vi "Flatten Multi D Arrays.vi"() -> ()   [LabVIEW 2011]
uses:
  JSON Scalar/variants/Variant Data Typdef.ctl
  <vilib>/Utility/VariantDataType/Type.ctl
  JSON Scalar/JSON Scalar.lvclass
  <vilib>/Utility/VariantDataType/VariantType.lvlib
panel:
  out "dimensions?":bool
  out "# 3D Array Dimensions":i32[](array[numeric])=[4, 3, 3]
  out "3D Variant Data":T1[](array[typedef])=[{"Type Enum"=enum."Double Float", "Name"="", "Variant"=variant(dbl 1.0)}, {"Type Enum"=enum."Double Float", "Name"="", "Variant"=variant(dbl 2.0)}, {"Type Enum"=enum."Double Float", "Name"="", "Variant"=variant(dbl 3.0)}, {"Type Enum"=enum."Double Float", "Name"="", "Variant"=variant(dbl 4.0)}, {"Type Enum"=enum."Double Float", "Name"="", "Variant"=variant(dbl 5.0)}, {"Type Enum"=enum."Double Float", "Name"="", "Variant"=variant(dbl 6.0)}, {"Type Enum"=enum."Double Float", "Name"="", "Variant"=variant(dbl 7.0)}, {"Type Enum"=enum."Double Float", "Name"="", "Variant"=variant(dbl 8.0)}, {"Type Enum"=enum."Double Float", "Name"="", "Variant"=variant(dbl 9.0)}, {"Type Enum"=enum."Double Float", "Name"="", "Variant"=variant(dbl 10.0)}, {"Type Enum"=enum."Double Float", "Name"="", "Variant"=variant(dbl 11.0)}, {"Type Enum"=enum."Double Float", "Name"="", "Variant"=variant(dbl 12.0)}, {"Type Enum"=enum."Double Float", "Name"="", "Variant"=variant(dbl 20.0)}, {"Type Enum"=enum."Double Float", "Name"="", "Variant"=variant(dbl 21.0)}, {"Type Enum"=enum."Double Float", "Name"="", "Variant"=variant(dbl 22.0)}, {"Type Enum"=enum."Double Float", "Name"="", "Variant"=variant(dbl 23.0)}, {"Type Enum"=enum."Double Float", "Name"="", "Variant"=variant(dbl 24.0)}, {"Type Enum"=enum."Double Float", "Name"="", "Variant"=variant(dbl 25.0)}, {"Type Enum"=enum."Double Float", "Name"="", "Variant"=variant(dbl 26.0)}, {"Type Enum"=enum."Double Float", "Name"="", "Variant"=variant(dbl 27.0)}, {"Type Enum"=enum."Double Float", "Name"="", "Variant"=variant(dbl 28.0)}, {"Type Enum"=enum."Double Float", "Name"="", "Variant"=variant(dbl 29.0)}, {"Type Enum"=enum."Double Float", "Name"="", "Variant"=variant(dbl 30.0)}, {"Type Enum"=enum."Double Float", "Name"="", "Variant"=variant(dbl 31.0)}, {"Type Enum"=enum."Double Float", "Name"="", "Variant"=variant(dbl 50.0)}, {"Type Enum"=enum."Double Float", "Name"="", "Variant"=variant(dbl 51.0)}, {"Type Enum"=enum."Double Float", "Name"="", "Variant"=variant(dbl 52.0)}, {"Type Enum"=enum."Double Float", "Name"="", "Variant"=variant(dbl 53.0)}, {"Type Enum"=enum."Double Float", "Name"="", "Variant"=variant(dbl 54.0)}, {"Type Enum"=enum."Double Float", "Name"="", "Variant"=variant(dbl 55.0)}, {"Type Enum"=enum."Double Float", "Name"="", "Variant"=variant(dbl 56.0)}, {"Type Enum"=enum."Double Float", "Name"="", "Variant"=variant(dbl 57.0)}, {"Type Enum"=enum."Double Float", "Name"="", "Variant"=variant(dbl 58.0)}, {"Type Enum"=enum."Double Float", "Name"="", "Variant"=variant(dbl 59.0)}, {"Type Enum"=enum."Double Float", "Name"="", "Variant"=variant(dbl 60.0)}, {"Type Enum"=enum."Double Float", "Name"="", "Variant"=variant(dbl 61.0)}]
  out "2D Variant Data":T1[](array[typedef])=[{"Type Enum"=enum."U64", "Name"="", "Variant"=variant(u64 1)}, {"Type Enum"=enum."U64", "Name"="", "Variant"=variant(u64 2)}, {"Type Enum"=enum."U64", "Name"="", "Variant"=variant(u64 3)}, {"Type Enum"=enum."U64", "Name"="", "Variant"=variant(u64 4)}, {"Type Enum"=enum."U64", "Name"="", "Variant"=variant(u64 5)}, {"Type Enum"=enum."U64", "Name"="", "Variant"=variant(u64 6)}, {"Type Enum"=enum."U64", "Name"="", "Variant"=variant(u64 7)}, {"Type Enum"=enum."U64", "Name"="", "Variant"=variant(u64 8)}, {"Type Enum"=enum."U64", "Name"="", "Variant"=variant(u64 9)}, {"Type Enum"=enum."U64", "Name"="", "Variant"=variant(u64 10)}, {"Type Enum"=enum."U64", "Name"="", "Variant"=variant(u64 11)}, {"Type Enum"=enum."U64", "Name"="", "Variant"=variant(u64 12)}]
  out "1D Variant Data":T1[](array[typedef])=[{"Type Enum"=enum."U8", "Name"="", "Variant"=variant(u8 1)}, {"Type Enum"=enum."U8", "Name"="", "Variant"=variant(u8 2)}, {"Type Enum"=enum."U8", "Name"="", "Variant"=variant(u8 3)}, {"Type Enum"=enum."U8", "Name"="", "Variant"=variant(u8 4)}]
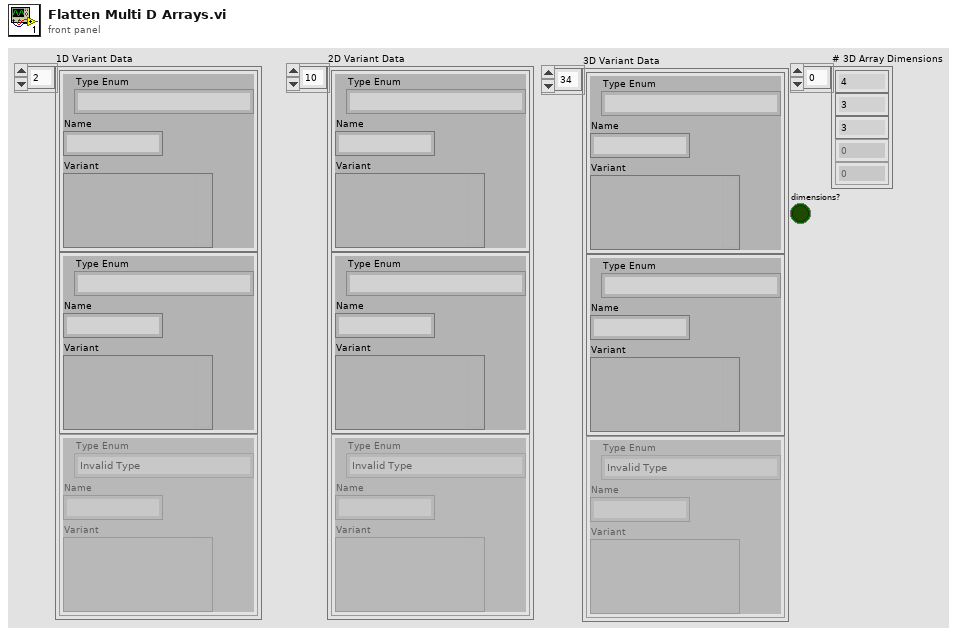
[diagram p1: front panel]
types:
  T1 = typedef "JSON Scalar.lvclass/Variant Data Typdef.ctl" = cluster{"Type Enum":T2, "Name":string, "Variant":variant}
  T2 = typedef "VariantType.lvlib/Type.ctl" = enum8{"Invalid Type", "Void", "I8", "I16", "I32", "I64", "U8", "U16", "U32", "U64", "Single Float", "Double Float", "Extended Float", "Single Complex", "Double Complex", "Extended Complex", "Enum U8", "Enum U16", "Enum U32", "Enum U64", "Single Float With Unit", "Double Float With Unit", "Extended Float With Unit", "Single Complex with Unit", "Double Complex with Unit", "Extended Complex with Unit", "Boolean", "String", "Path", "Picture", "Tag", "Array", "Cluster", "Variant", "LV Variant", "Waveform", "Timestamp", "Digital Waveform", "Digital Data", "ExpressData", "Refnum", "External Data", "VI", "Poly VI", "LabVIEW Class Instance", "Fixed Point"}
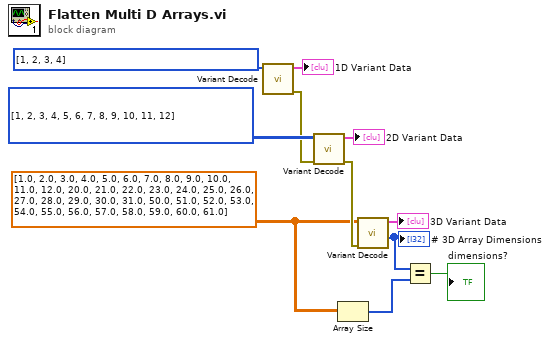
[diagram p0: block diagram]
diagram:
  w4 = dbl[][][] [[[1.0, 2.0, 3.0, 4.0], [5.0, 6.0, 7.0, 8.0], [9.0, 10.0, 11.0, 12.0]], [[20.0, 21.0, 22.0, 23.0], [24.0, 25.0, 26.0, 27.0], [28.0, 29.0, 30.0, 31.0]], [[50.0, 51.0, 52.0, 53.0], [54.0, 55.0, 56.0, 57.0], [58.0, 59.0, 60.0, 61.0]]]
  n1 = call "Variant Decode.vi"("variant"=u8[] [1, 2, 3, 4]) -> ("error out"=w6:errorcluster, "Variant Data"=→"1D Variant Data":T1[])  [unwired: 8 in, 1 out]
  n2 = call "Variant Decode.vi"("error in (no error)"=w6, "variant"=u64[][] [[1, 2, 3, 4], [5, 6, 7, 8], [9, 10, 11, 12]]) -> ("error out"=w5:errorcluster, "Variant Data"=→"2D Variant Data":T1[])  [unwired: 7 in, 1 out]
  n3 = Array Size(array=w4) -> (size(s)=w2:i32[])
  n4 = call "Variant Decode.vi"("error in (no error)"=w5, "variant"=w4) -> ("Array Dimensions (Reversed)"=w3:i32[], "Variant Data"=→"3D Variant Data":T1[])  [unwired: 7 in, 1 out]
  "# 3D Array Dimensions" <- w3
  n5 = Equal?(x=w3, y=w2) -> (x = y?=→"dimensions?":bool)
